vi "RS_RF_send_command_LAN.vi"(1 "Value":dbl=3.0, 2 "Parameter":T1(ring), 3 "IP Address":string="192.168.0.21") -> ()   [LabVIEW 2013]
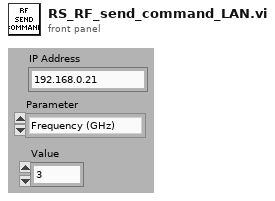
[diagram p1: front panel]
types:
  T1 = enum16{"Frequency (GHz)", "Power (dBm)", "Pulse period (us)", "Pulse width (us)", "Pulse delay (us)", "Pulse modulation?", "Output on?", "Pulse source", "Pulse mode", "Trigger mode", "Ex trigger input slope", "External impedance"}
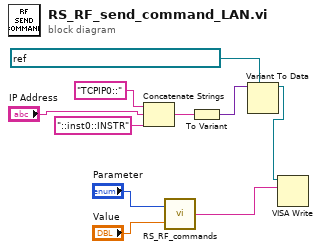
[diagram p0: block diagram]
diagram:
  n1 = Concatenate Strings("TCPIP0::" ("string"), "IP Address", "::inst0::INSTR" ("string")) -> (w7:string)
  n2 = call "RS_RF_commands.vi"("Value"="Value", "Parameter"="Parameter") -> ("Command"=w8:string)
  n3 = To Variant(anything=w7) -> (Variant=w4:variant)
  n4 = Variant To Data(type=refnum<visa-resource-name> "TCPIP0::192.168.137.3::inst0::INSTR" ("VISA resource name"), Variant=w4) -> (data=w1:refnum<visa-resource-name>)  [unwired: 1 in, 1 out]
  n5 = VISA Write(VISA resource name=w1, write buffer=w8) -> ()  [unwired: 1 in, 3 out]
